vi "XImc Example Three axes.vi"() -> ()   [LabVIEW 2012]
uses:
  subvi/XImc Example 1 CS.ctl
  libximc.lvlib
panel:
  out "s/n 3":u32
  out "s/n 2":u32
  out "s/n 1":u32
  in  "Destination 6":i32
  in  "Destination 5":i32
  in  "Destination 4":i32
  in  "Start shift":bool
  in  "Destination 3":i32
  in  "Destination 2":i32
  out "Cur pos 3":dbl format="%#.2f"
  out "Cur pos 2":dbl format="%#.2f"
  in  "Controller 3":u16(ring) items=["\\\\.\\COM10", "\\\\.\\COM9", "\\\\.\\COM7"]
  in  "Controller 2":u16(ring) items=["\\\\.\\COM10", "\\\\.\\COM9", "\\\\.\\COM7"]
  in  "Stop motion":bool
  in  "Start move":bool
  in  "Destination 1":i32
  out "Cur pos 1":dbl format="%#.2f"
  in  "Controller 1":u16(ring) items=["\\\\.\\COM10", "\\\\.\\COM9", "\\\\.\\COM7"]
  in  "Find controllers":bool
  in  "Close application":bool
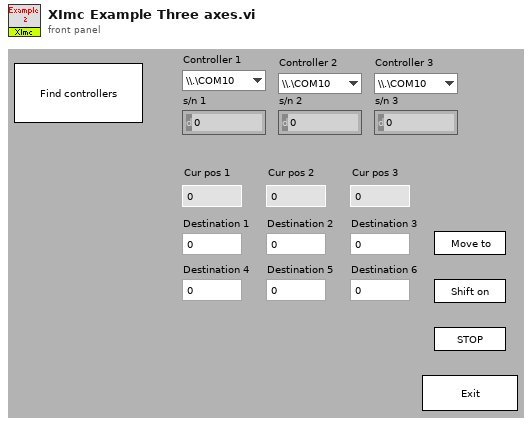
[diagram p1: front panel]
types:
  T1 = typedef "XImc Example 1 CS.ctl" = enum16{"Initialize_App", "Idle", "Find_Controllers", "Initialize_Controller", "Set_Parameters", "Get_Status", "Start_Motion", "Move_Relative", "Stop_Motion", "ZEROCOMM", "HOME", "LEFT", "RIGT", "SSTP", "Close_Controller", "Error_Handler", "Close_App", "Get_Move_Settings", "Set_Move_Settings"}
  T2 = cluster{"Number of controllers":i32, "Controllers' names":string[], "variant":variant, "quit":bool, "IDs":i32[]}
  T3 = cluster{"Destination 4":i32, "Destination 5":i32, "Destination 6":i32}
  T4 = cluster{"Destination 1":i32, "Destination 2":i32, "Destination 3":i32}
  T5 = cluster{"MoveSts":u32, "MvCmdSts":u32, "PWRSts":u32, "EncSts":u32, "WindSts":u32, "CurPosition":i32, "uCurPosition":i32, "@dummy control@":i8, "@dummy control@":i8, "@dummy control@":i8, "@dummy control@":i8, "EncPosition":i64, "CurSpeed":i32, "uCurSpeed":i32, "Ipwr":i32, "Upwr":i32, "Iusb":i32, "Uusb":i32, "CurT":i32, "Flags":u32, "GPIOFlags":u32, "CmdBufFreeSpace":u32}
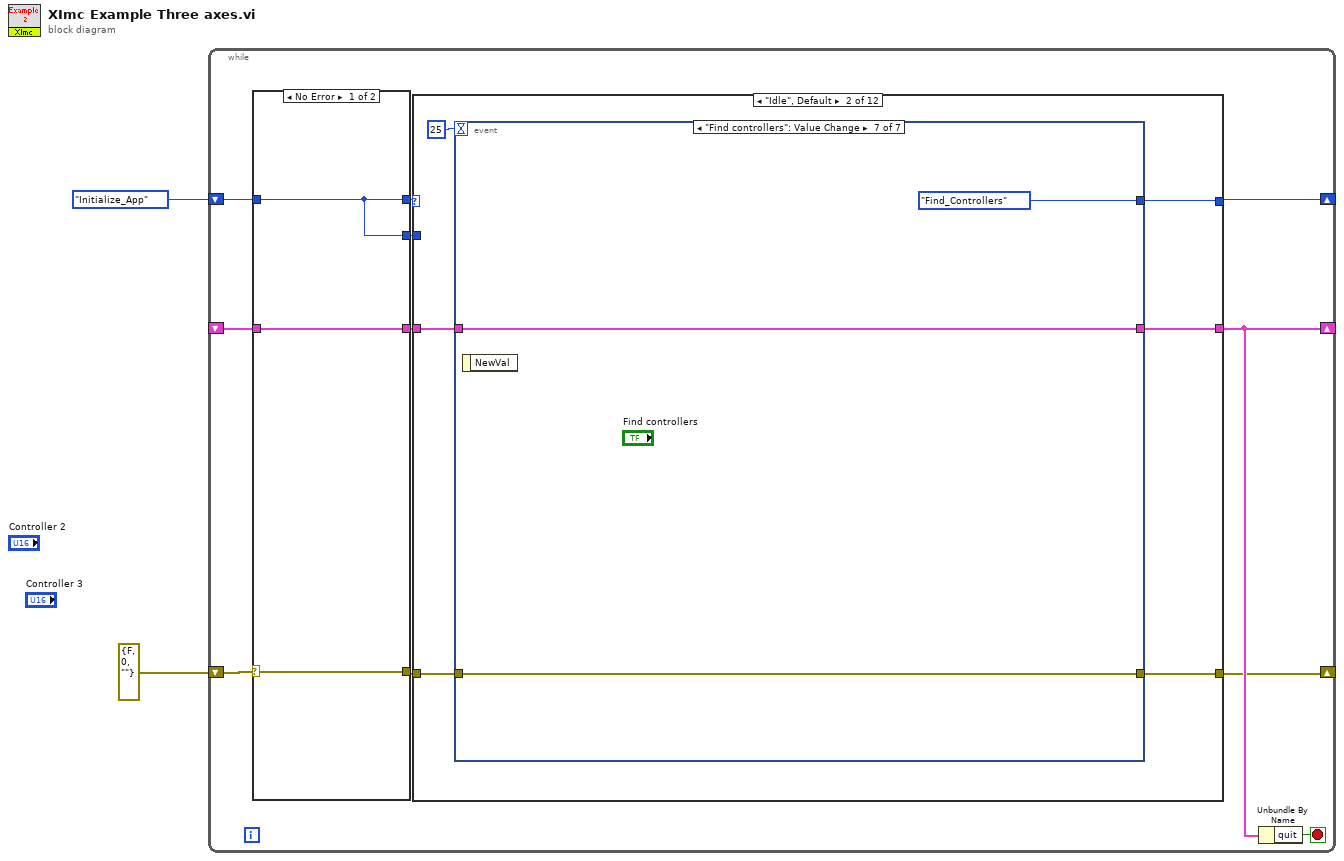
[diagram p0: block diagram]
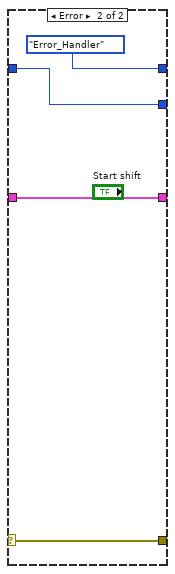
[diagram p2: hidden frame]
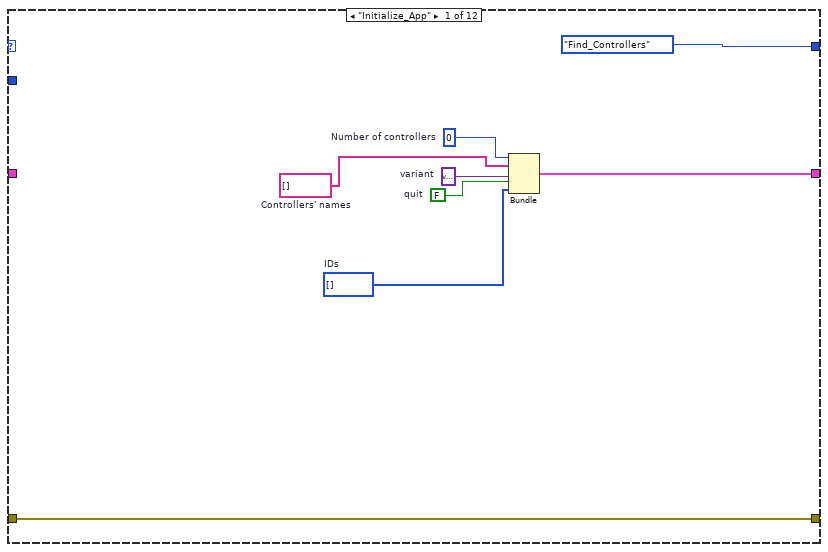
[diagram p3: hidden frame]
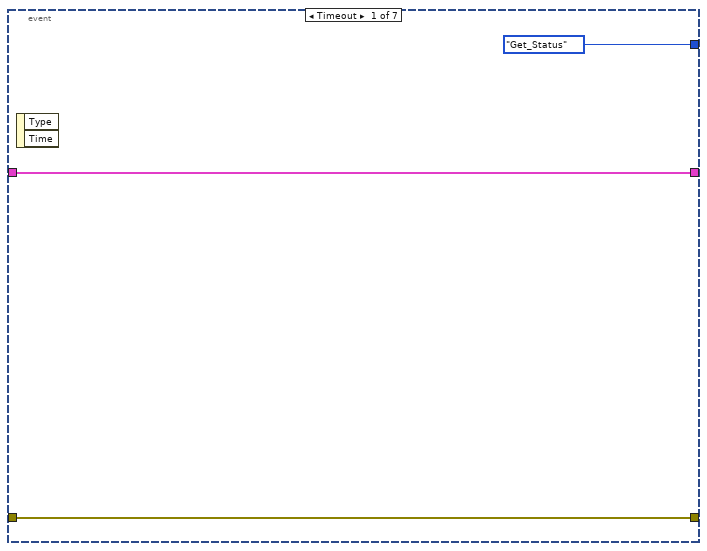
[diagram p4: hidden frame]
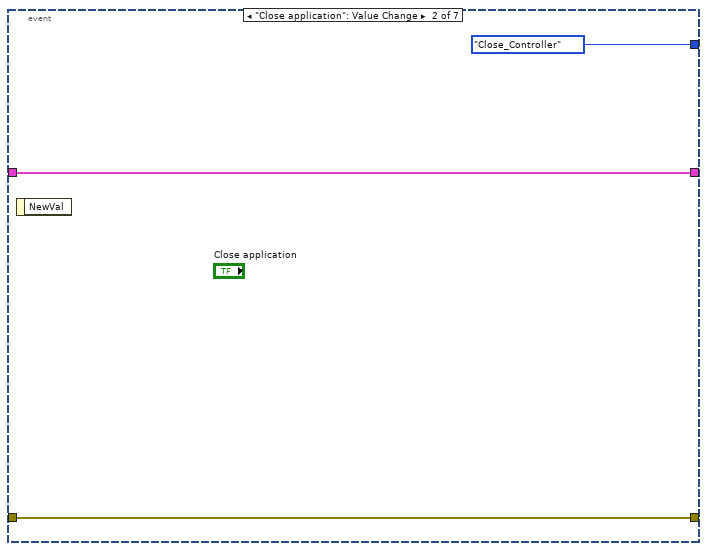
[diagram p5: hidden frame]
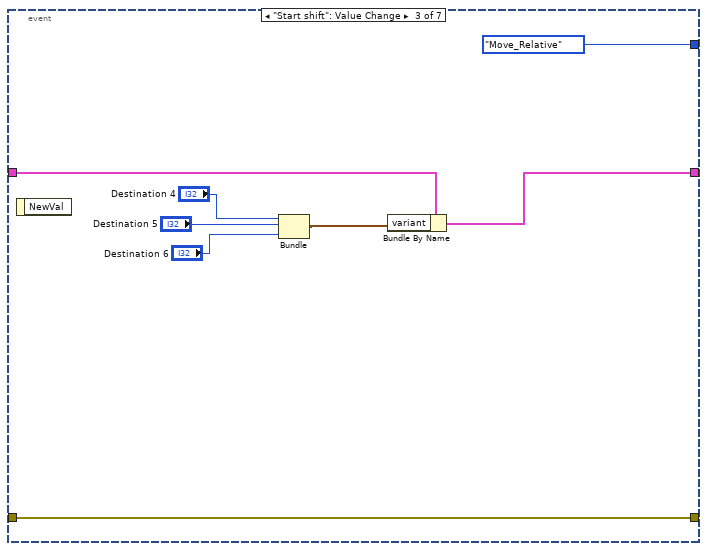
[diagram p6: hidden frame]
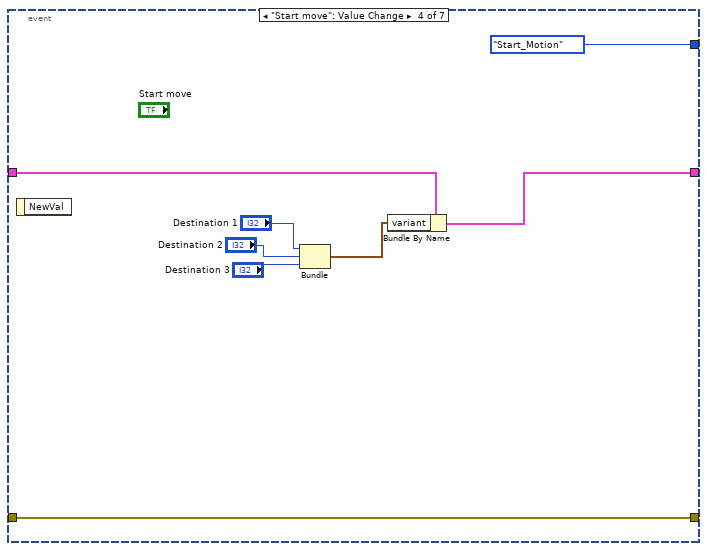
[diagram p7: hidden frame]
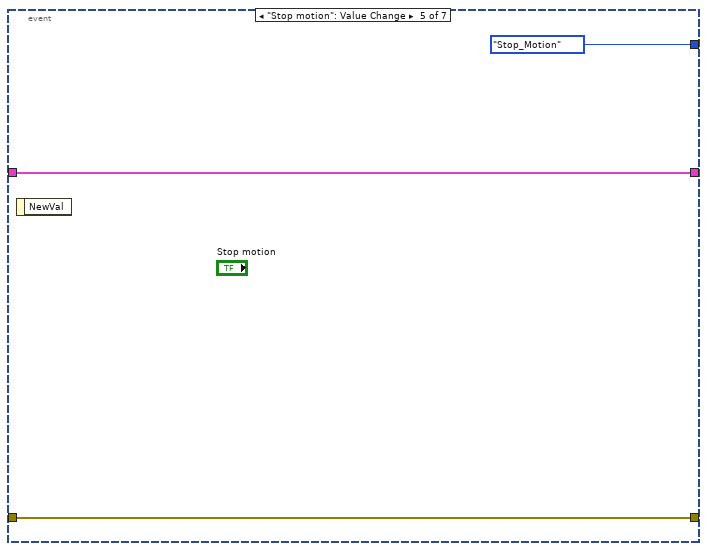
[diagram p8: hidden frame]
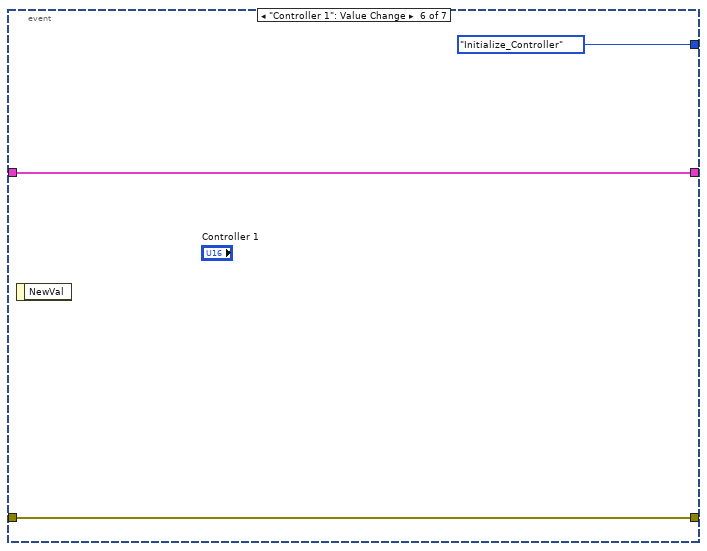
[diagram p9: hidden frame]
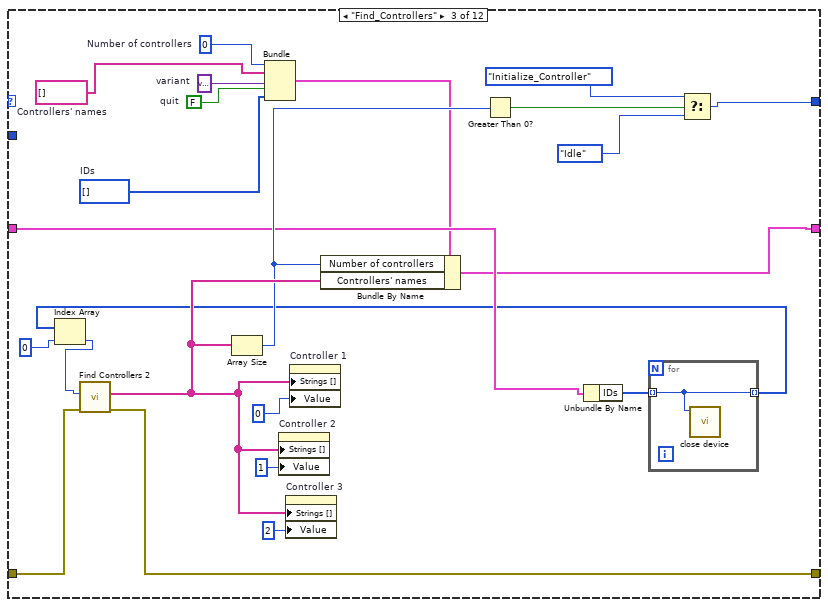
[diagram p10: hidden frame]
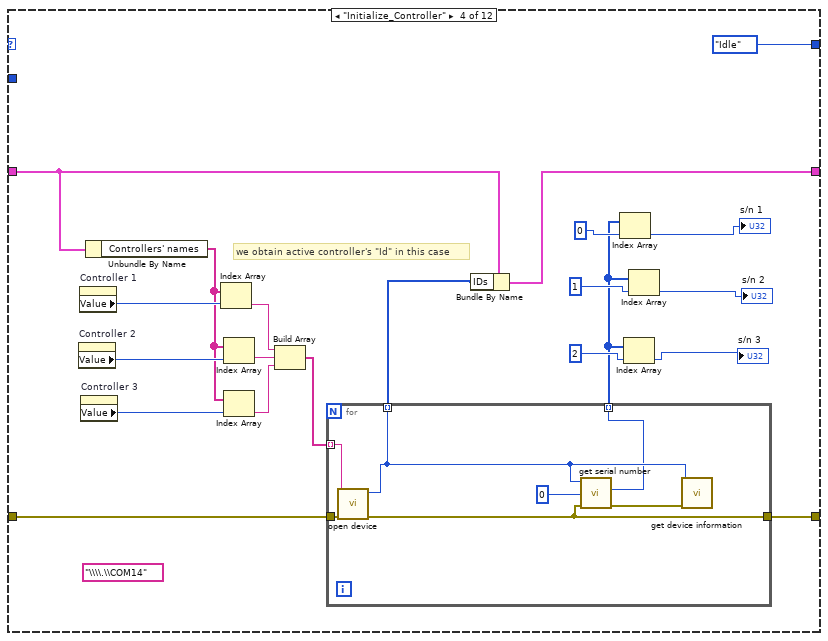
[diagram p11: hidden frame]
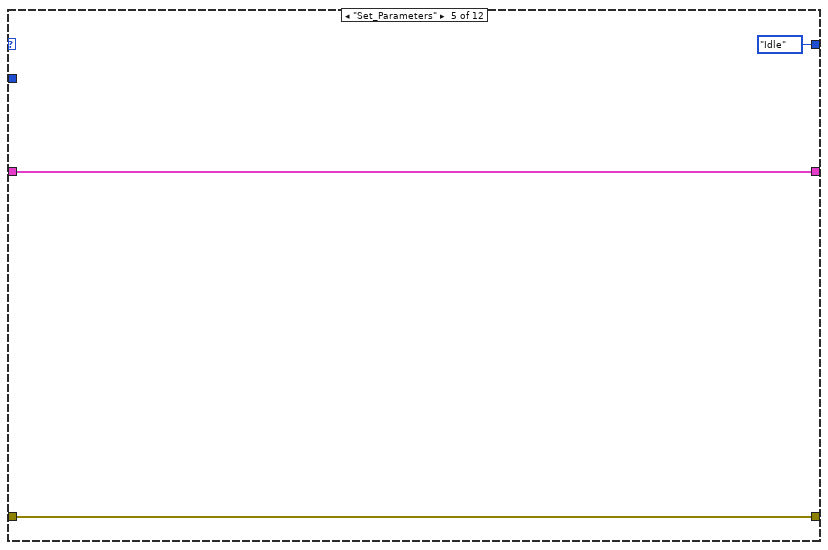
[diagram p12: hidden frame]
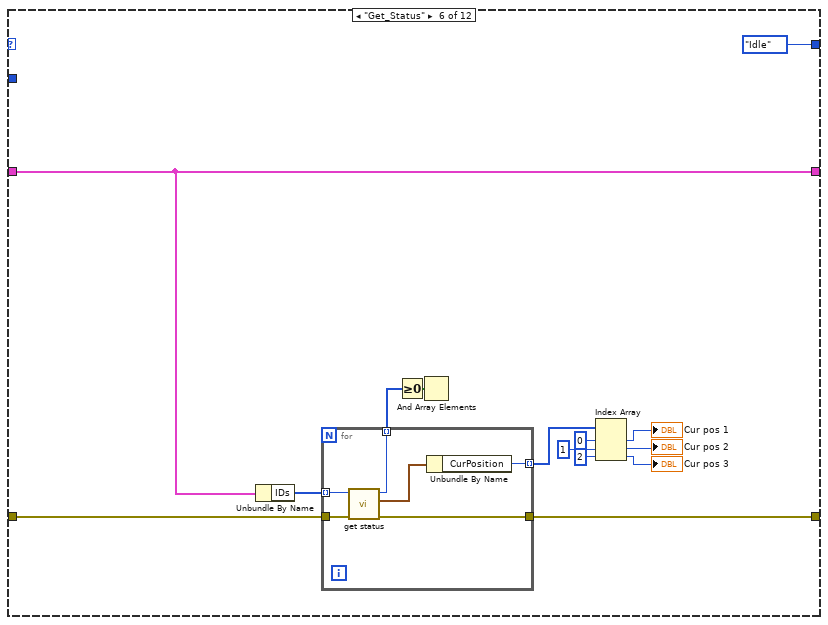
[diagram p13: hidden frame]
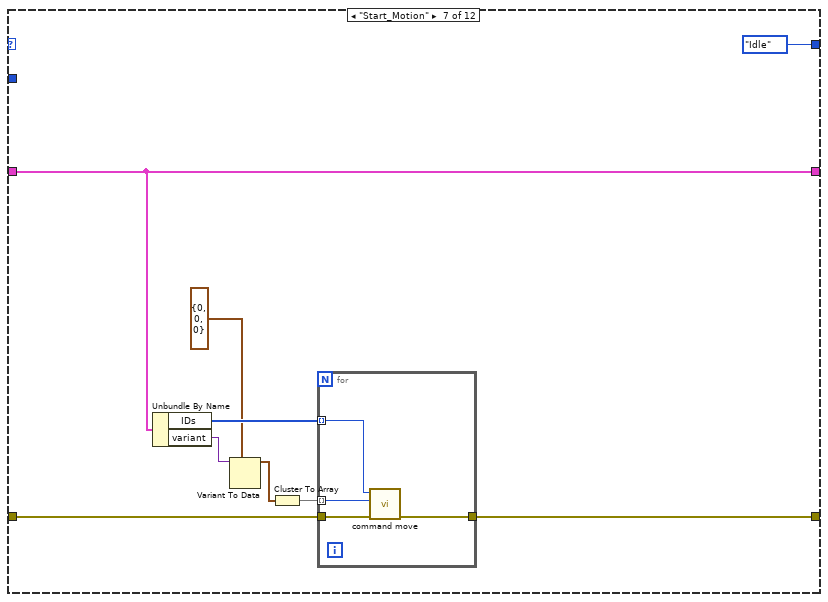
[diagram p14: hidden frame]
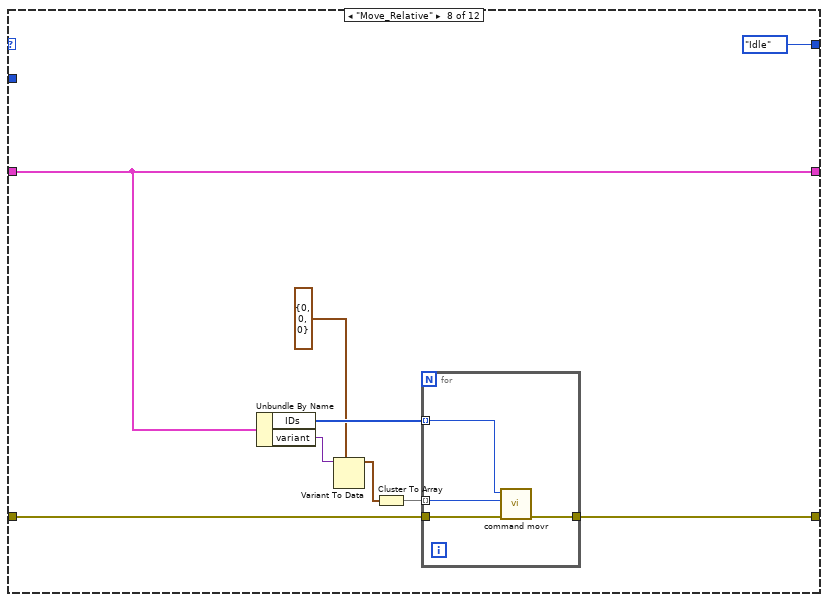
[diagram p15: hidden frame]
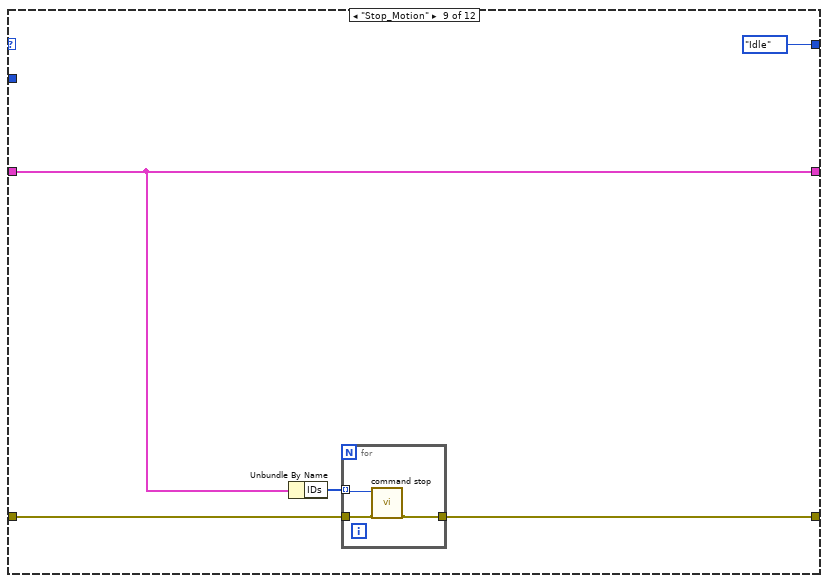
[diagram p16: hidden frame]
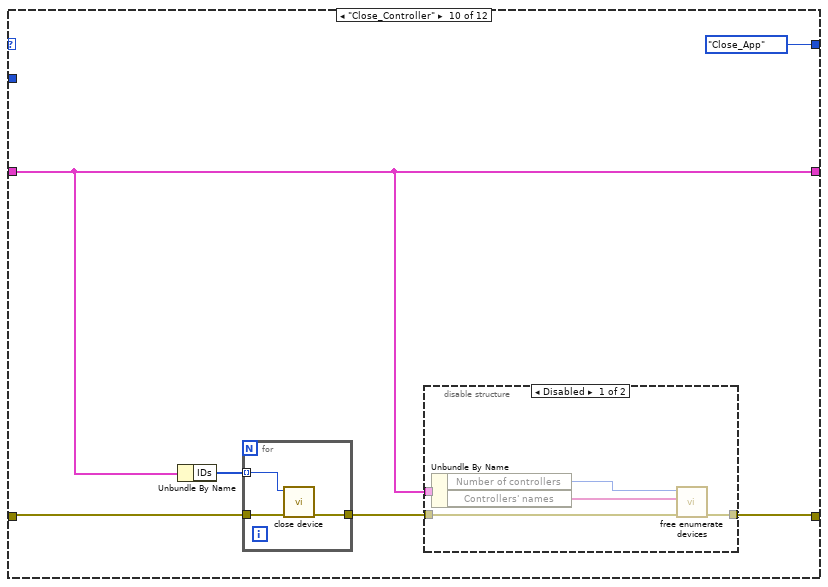
[diagram p17: hidden frame]
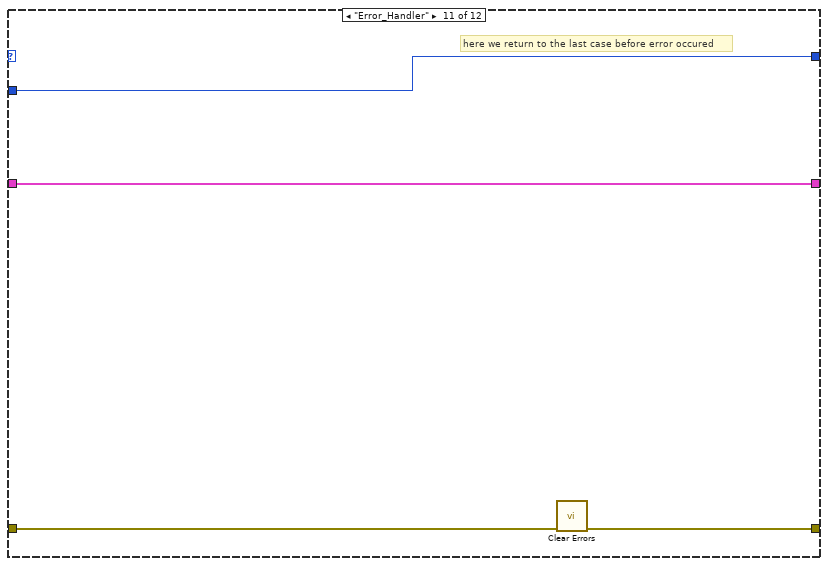
[diagram p19: hidden frame]
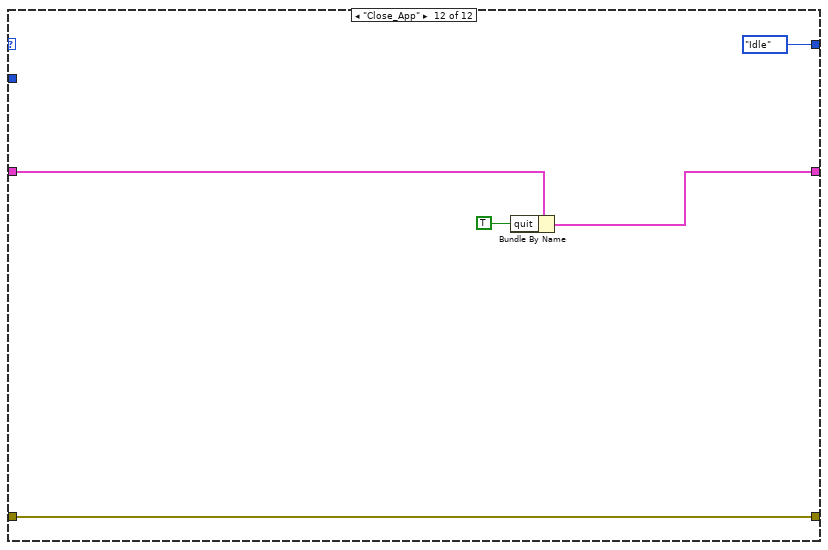
[diagram p20: hidden frame]
diagram:
  n1 = while {
    shift-right: [w13] -> _
    shift-left: XImc_Example_1_CS."Initialize_App" ("Case") -> [w7]
    shift-right: [w12] -> _
    shift-left: _ -> [w9]
    shift-right: [w4] -> _
    shift-left: errorcluster {"status"=FALSE, "code"=0, "source"=""} ("error in (no error)") -> [w11]
    stop <- w3 stop-if-true
    n2 = case shown="No Error" w11 {
      selector: w11 -> [w16 w19]
      tunnel: [w16 w19] -> w10
      tunnel: w9 -> [w15 w17]
      tunnel: [w15 w17] -> w8
      tunnel: w7 -> [w14 w18]
      tunnel: [w14 XImc_Example_1_CS."Error_Handler" ("Case")] -> w6
      tunnel: [w14 w18] -> w5
      frame No Error {
      }
      frame Error {
      }
    }
    n3 = case shown="\"Idle\", Default" w6 {
      tunnel: [XImc_Example_1_CS."Find_Controllers" ("Case") w32 w86 XImc_Example_1_CS."Idle" ("Case") XImc_Example_1_CS."Idle" ("Case") XImc_Example_1_CS."Idle" ("Case") XImc_Example_1_CS."Idle" ("Case") XImc_Example_1_CS."Idle" ("Case") XImc_Example_1_CS."Idle" ("Case") XImc_Example_1_CS."Close_App" ("Case") w192 XImc_Example_1_CS."Idle" ("Case")] -> w13
      tunnel: [w21 w31 w71 w107 w119 w131 w148 w155 w170 w177 w191 w194] -> w12
      tunnel: w10 -> [w25 w34 w67 w108 w118 w133 w147 w157 w169 w176 w190 w197]
      tunnel: w8 -> [_ w30 w78 w102 w119 w131 w148 w155 w170 w177 w191 w195]
      tunnel: w5 -> [_ _ _ _ _ _ _ _ _ _ w192 _]
      tunnel: [w25 w29 w66 w106 w118 w132 w146 w156 w167 w178 w189 w197] -> w4
      frame "Initialize_App" {
        w22 = i32[] []  # IDs
        w23 = string[] []  # Controllers' names
        w24 = 0  # Number of controllers
        w26 = FALSE  # quit
        w27 = variant  # variant
        n4 = Bundle("Number of controllers"=w24, "Controllers' names"=w23, "variant"=w27, "quit"=w26, "IDs"=w22) -> (w21:T2)  [unwired: 1 in]
      }
      frame "Idle", Default {
        n5 = event shown="[6] \"Find controllers\": Value Change" {
          selector: _ -> [_ _ _ _ _ _ _]
          dyn-events: _ -> [_ _ _ _ _ _ _]
          timeout: 25 -> [_ _ _ _ _ _ _]
          tunnel: w34 -> [w35 w38 w47 w55 w58 w61 w63]
          tunnel: [XImc_Example_1_CS."Get_Status" ("Case") XImc_Example_1_CS."Close_Controller" ("Case") XImc_Example_1_CS."Move_Relative" ("Case") XImc_Example_1_CS."Start_Motion" ("Case") XImc_Example_1_CS."Stop_Motion" ("Case") XImc_Example_1_CS."Initialize_Controller" ("Case") XImc_Example_1_CS."Find_Controllers" ("Case")] -> w32
          tunnel: [w36 w39 w45 w53 w57 w60 w64] -> w31
          tunnel: w30 -> [w36 w39 w46 w54 w57 w60 w64]
          tunnel: [w35 w38 w47 w55 w58 w61 w63] -> w29
          event Timeout {
            n6 = event-data() -> ()  [unwired: 1 in, 2 out]
          }
          event "Close application": Value Change {
            n7 = event-data() -> ()  [unwired: 1 in, 1 out]
          }
          event "Start shift": Value Change {
            n8 = event-data() -> ()  [unwired: 1 in, 1 out]
            n9 = Bundle("Destination 4"="Destination 4", "Destination 5"="Destination 5", "Destination 6"="Destination 6") -> (w44:T3)  [unwired: 1 in]
            n10 = Bundle By Name(cluster=w46, "variant"=w44) -> (w45:T2)
          }
          event "Start move": Value Change {
            n11 = event-data() -> ()  [unwired: 1 in, 1 out]
            n12 = Bundle("Destination 1"="Destination 1", "Destination 2"="Destination 2", "Destination 3"="Destination 3") -> (w49:T4)  [unwired: 1 in]
            n13 = Bundle By Name(cluster=w54, "variant"=w49) -> (w53:T2)
          }
          event "Stop motion": Value Change {
            n14 = event-data() -> ()  [unwired: 1 in, 1 out]
          }
          event "Controller 1": Value Change {
            n15 = event-data() -> ()  [unwired: 1 in, 1 out]
          }
          event "Find controllers": Value Change {
            n16 = event-data() -> ()  [unwired: 1 in, 1 out]
          }
        }
      }
      frame "Find_Controllers" {
        w73 = i32[] []  # IDs
        w74 = string[] []  # Controllers' names
        w75 = 0  # Number of controllers
        w76 = FALSE  # quit
        w77 = variant  # variant
        n17 = Bundle("Number of controllers"=w75, "Controllers' names"=w74, "variant"=w77, "quit"=w76, "IDs"=w73) -> (w72:T2)  [unwired: 1 in]
        n18 = Unbundle By Name(w78) -> ("IDs"=w79:i32[])
        n19 = for {
          tunnel: w79 -> [w89] mode=indexing
          tunnel: [w89] -> w70 mode=indexing
          n20 = call "close device.vi"("id"=w89) -> ()  [unwired: 8 in, 3 out]
        }
        n21 = Index Array(array=w70, index=0) -> (element=w69:i32)
        n22 = call "Find Controllers 2.vi"("error in (no error)"=w67, "Numeric"=w69) -> ("error out"=w66:errorcluster, "Names"=w81:string[])  [unwired: 8 in]
        n23 = Array Size(array=w81) -> (size(s)=w80:i32)
        n24 = property on="Controller 2" class="Ring (strict)"("Strings []"=w81, "Value"=1) -> ()  [unwired: 2 in, 2 out]
        n25 = property on="Controller 3" class="Ring (strict)"("Strings []"=w81, "Value"=2) -> ()  [unwired: 2 in, 2 out]
        n26 = property on="Controller 1" class="Ring (strict)"("Strings []"=w81, "Value"=0) -> ()  [unwired: 2 in, 2 out]
        n27 = Bundle By Name(cluster=w72, "Number of controllers"=w80, "Controllers' names"=w81) -> (w71:T2)
        n28 = Greater Than 0?(x=w80) -> (x > 0?=w88:bool)
        n29 = Select(t=XImc_Example_1_CS."Initialize_Controller", s=w88, f=XImc_Example_1_CS."Idle" ("Case")) -> (s? t:f=w86:T1)
      }
      frame "Initialize_Controller" {
        (unwired) "\\\\.\\COM14" ("name")
        # "we obtain active controller's \"Id\" in this case"
        n30 = property on="Controller 2" class="Ring (strict)"() -> ("Value"=w104:u16)  [unwired: 2 in, 2 out]
        n31 = property on="Controller 1" class="Ring (strict)"() -> ("Value"=w109:u16)  [unwired: 2 in, 2 out]
        n32 = property on="Controller 3" class="Ring (strict)"() -> ("Value"=w103:u16)  [unwired: 2 in, 2 out]
        n33 = Unbundle By Name(w102) -> ("Controllers' names"=w97:string[])
        n34 = Index Array(array=w97, index=w109) -> (element=w99:string)
        n35 = Index Array(array=w97, index=w104) -> (element=w100:string)
        n36 = Index Array(array=w97, index=w103) -> (element=w101:string)
        n37 = Build Array(w99, w100, w101) -> (w98:string[])
        n38 = for {
          tunnel: w108 -> [w117]
          tunnel: [w113] -> w106
          tunnel: [w114] -> w105 mode=indexing
          tunnel: w98 -> [w112] mode=indexing
          tunnel: [w111] -> w93 mode=indexing
          n39 = call "open device.vi"("error in (no error)"=w117, "name"=w112) -> ("error out"=w113:errorcluster, "function return"=w114:i32)  [unwired: 8 in]
          n40 = call "get serial number.vi"("error in (no error)"=w113, "SerialNumber"=u32 0 ("serial"), "id"=w114) -> ("error out"=w115:errorcluster, "SerialNumber out"=w111:u32)  [unwired: 6 in, 1 out]
          n41 = call "get device information.vi"("error in (no error)"=w115, "id"=w114) -> ()  [unwired: 7 in, 3 out]
        }
        n42 = Bundle By Name(cluster=w102, "IDs"=w105) -> (w107:T2)
        n43 = Index Array(array=w93, index=u32 0 ("serial")) -> (element=→"s/n 1":u32)
        n44 = Index Array(array=w93, index=u32 2 ("serial")) -> (element=→"s/n 3":u32)
        n45 = Index Array(array=w93, index=u32 1 ("serial")) -> (element=→"s/n 2":u32)
      }
      frame "Set_Parameters" {
      }
      frame "Get_Status" {
        n46 = Unbundle By Name(w131) -> ("IDs"=w130:i32[])
        n47 = for {
          tunnel: w133 -> [w140]
          tunnel: [w139] -> w132
          tunnel: [w138] -> w128 mode=indexing
          tunnel: w130 -> [w135] mode=indexing
          tunnel: [w137] -> w129 mode=indexing
          n48 = call "get status.vi"("error in (no error)"=w140, "id"=w135) -> ("error out"=w139:errorcluster, "status out"=w136:T5, "function return"=w137:i32)  [unwired: 7 in]
          n49 = Unbundle By Name(w136) -> ("CurPosition"=w138:i32)
        }
        n50 = Greater Or Equal To 0?(x=w129) -> (x >= 0?=w121:bool[])
        n51 = And Array Elements(Boolean array=w121) -> ()  [unwired: 1 out]
        n52 = Index Array(array=w128, index #1=0 ("index"), index #2=1 ("index"), index #3=2 ("index")) -> (element #1=→"Cur pos 1":i32, element #2=→"Cur pos 2":i32, element #3=→"Cur pos 3":i32)
      }
      frame "Start_Motion" {
        n53 = Unbundle By Name(w148) -> ("IDs"=w144:i32[], "variant"=w141:variant)
        n54 = Variant To Data(type=cluster{u32, u32, u32} {0, 0, 0}, Variant=w141) -> (data=w145:cluster{u32, u32, u32})  [unwired: 1 in, 1 out]
        n55 = Cluster To Array(cluster=w145) -> (array=w142:u32[])
        n56 = for {
          tunnel: w147 -> [w153]
          tunnel: [w152] -> w146
          tunnel: w142 -> [w151] mode=indexing
          tunnel: w144 -> [w150] mode=indexing
          n57 = call "command move.vi"("error in (no error)"=w153, "Position"=w151, "id"=w150) -> ("error out"=w152:errorcluster)  [unwired: 7 in, 1 out]
        }
      }
      frame "Move_Relative" {
        n58 = Unbundle By Name(w155) -> ("IDs"=w160:i32[], "variant"=w154:variant)
        n59 = Variant To Data(type=cluster{u32, u32, u32} {0, 0, 0}, Variant=w154) -> (data=w161:cluster{u32, u32, u32})  [unwired: 1 in, 1 out]
        n60 = Cluster To Array(cluster=w161) -> (array=w158:u32[])
        n61 = for {
          tunnel: w157 -> [w165]
          tunnel: [w164] -> w156
          tunnel: w158 -> [w166] mode=indexing
          tunnel: w160 -> [w163] mode=indexing
          n62 = call "command movr.vi"("error in (no error)"=w165, "DeltaPosition"=w166, "id"=w163) -> ("error out"=w164:errorcluster)  [unwired: 7 in, 1 out]
        }
      }
      frame "Stop_Motion" {
        n63 = Unbundle By Name(w170) -> ("IDs"=w168:i32[])
        n64 = for {
          tunnel: w169 -> [w174]
          tunnel: w168 -> [w172] mode=indexing
          tunnel: [w173] -> w167
          n65 = call "command stop.vi"("error in (no error)"=w174, "id"=w172) -> ("error out"=w173:errorcluster)  [unwired: 8 in, 1 out]
        }
      }
      frame "Close_Controller" {
        n66 = Unbundle By Name(w177) -> ("IDs"=w175:i32[])
        n67 = for {
          tunnel: [w183] -> w179
          tunnel: w176 -> [w182]
          tunnel: w175 -> [w181] mode=indexing
          n68 = call "close device.vi"("error in (no error)"=w182, "id"=w181) -> ("error out"=w183:errorcluster)  [unwired: 7 in, 2 out]
        }
        n69 = disable-structure shown="Disabled" {
          disable-tunnel: w179 -> [w188 _]
          disable-tunnel: [w187 _] -> w178
          disable-tunnel: w177 -> [w186 _]
          frame Disabled {
            n70 = Unbundle By Name(w186) -> ("Number of controllers"=w185:i32, "Controllers' names"=w184:string[])
            n71 = call "free enumerate devices.vi"("error in (no error)"=w188, 10:w184, "device_enumeration"=w185) -> ("error out"=w187:errorcluster)  [unwired: 7 in, 1 out]
          }
          frame Enabled {
          }
        }
      }
      frame "Error_Handler" {
        # "here we return to the last case before error occured"
        n72 = call <vilib>:"Clear Errors.vi"("error in (no error)"=w190) -> ("error out"=w189:errorcluster)  [unwired: 6 in]
      }
      frame "Close_App" {
        n73 = Bundle By Name(cluster=w195, "quit"=TRUE) -> (w194:T2)
      }
    }
    n74 = Unbundle By Name(w12) -> ("quit"=w3:bool)
  }
